vi "写入起始坐标.vi"(8 "error in (no error)":errorcluster caption="错误输入（无错误）", 10 "起始坐标":cluster{"Horizontal":i32, "Vertical":i32}, 11 "程序输入":refnum<class "程序.lvclass">) -> (0 "error out":errorcluster caption="错误输出", 3 "程序输出":refnum<class "程序.lvclass">)   [LabVIEW 2020, in "程序.lvclass"]
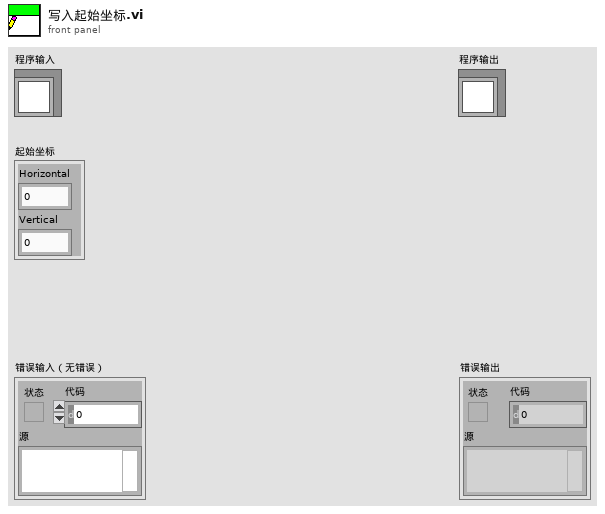
[diagram p1: front panel]
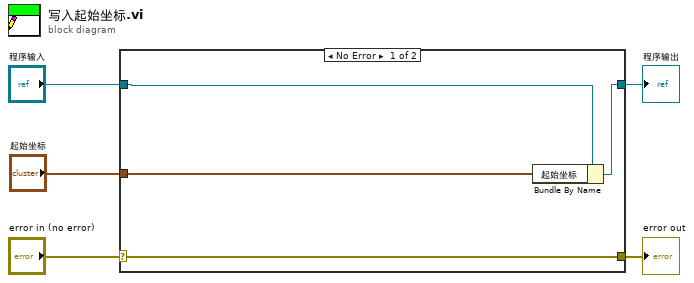
[diagram p0: block diagram]
diagram:
  n1 = case shown="No Error" "error in (no error)" {
    selector: "error in (no error)" -> [w9 w10]
    tunnel: [w9 w10] -> w4
    tunnel: [w8 w11] -> w2
    tunnel: "程序输入" -> [w7 w11]
    tunnel: "起始坐标" -> [w6 _]
    frame No Error {
      n2 = Bundle By Name(cluster=w7, "起始坐标"=w6) -> (w8:refnum<class "程序.lvclass">)
    }
    frame Error {
    }
  }
  "error out" <- w4
  "程序输出" <- w2
